vi "Pre Launch Init.vi"(11 "Connecting in":refnum<class "Connecting.lvclass">) -> (0 "error out":errorcluster, 3 "Connecting out":refnum<class "Connecting.lvclass">)   [LabVIEW 2013, in "Receiver.lvlib" / "ReceiverStates.lvlib" / "Connecting.lvclass"]
doc: "(<B>Filename</B>: Actor Framework.lvlib:Actor.lvclass:Pre Launch Init.vi)\n\nDefines behavior that occurs after the Launch Actor method is invoked but before the actor's Actor Core method begins running.\n\nThe Pre Launch Init method is guaranteed to finish before the Launch Actor method returns to its caller and before the actor itself receives any messages. Any references that the Pre Launch Init method obtains are guaranteed to have the same lifetime as the actor itself. Any errors that the Pre Launch Init method returns will abort the launch.\n\nBy default, this method does nothing. A descendant class may override it to define behavior."
uses:
  Connecting.lvclass
  ReceiverState/ReceiverState.lvclass
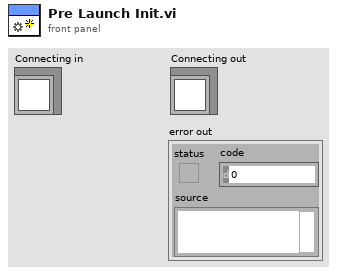
[diagram p1: front panel]
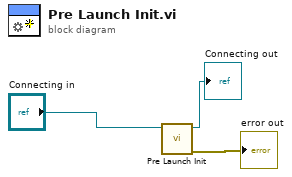
[diagram p0: block diagram]
diagram:
  n1 = call-parent "Pre Launch Init.vi"("ReceiverState in"="Connecting in") -> ("error out"=→"error out":errorcluster, "ReceiverState out"=→"Connecting out":refnum<class "Connecting.lvclass">)  [unwired: 9 in]
